vi "insert.vi"(8 "error in (no error)":errorcluster, 9 "Value":variant, 10 "Key":string, 11 "HashMap in":refnum<class "HashMap.lvclass">) -> (0 "error out":errorcluster, 3 "HashMap out":refnum<class "HashMap.lvclass">)   [LabVIEW 2017, in "HashMap.lvclass"]
uses:
  <userlib>/836-Library/Data_Structures/HashMap/HashMap.lvclass
  <userlib>/836-Library/Data_Structures/HashMap/HashMap.lvclass/HashMap.ctl
  <userlib>/836-Library/Data_Structures/Bucket/Types/KeyValuePair.ctl
  <vilib>/Utility/error.llb/Error Cluster From Error Code.vi
  <vilib>/ErrorRing/Error Ring.xnode
  <userlib>/836-Library/Data_Structures/Bucket/Bucket.lvclass
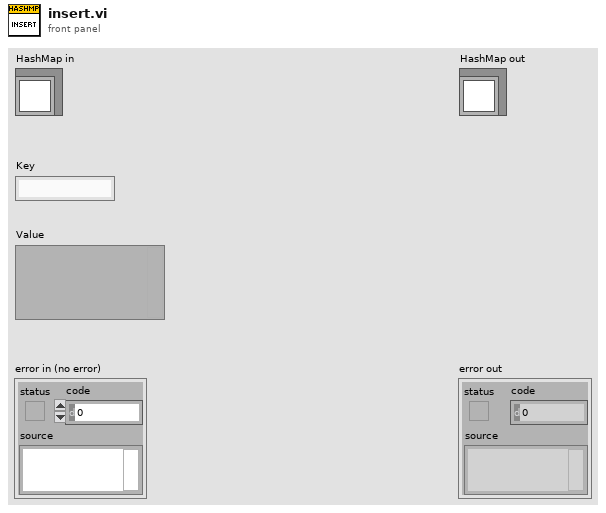
[diagram p1: front panel]
types:
  T1 = typedef "KeyValuePair.ctl" = cluster{"Key":string, "Value":variant}
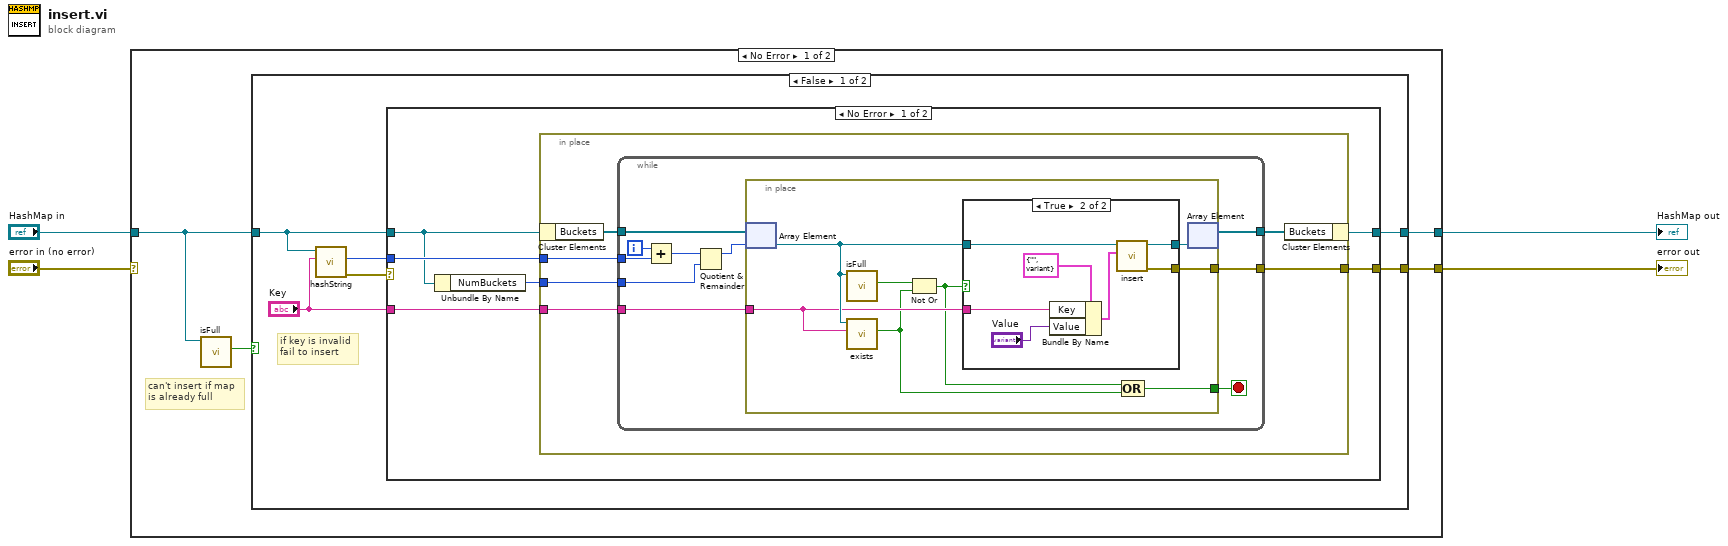
[diagram p0: block diagram]
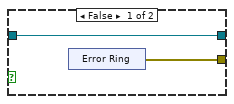
[diagram p2: hidden frame]
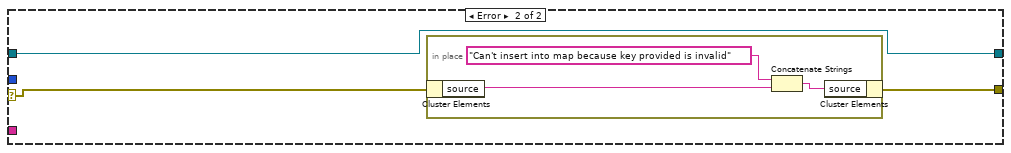
[diagram p3: hidden frame]
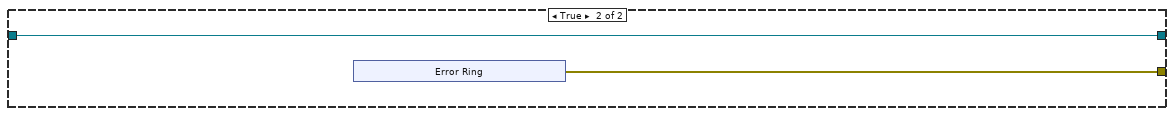
[diagram p4: hidden frame]
diagram:
  n1 = case shown="No Error" "error in (no error)" {
    selector: "error in (no error)" -> [_ w69]
    tunnel: [w6 w69] -> w3
    tunnel: [w5 w68] -> w1
    tunnel: "HashMap in" -> [w7 w68]
    frame No Error {
      # "can't insert if map\nis already full"
      n2 = call <userlib>:"isFull.vi"("HashMap in"=w7) -> ("Full?"=w8:bool)  [unwired: 8 in, 2 out]
      n3 = case shown="False" w8 {
        tunnel: w7 -> [w14 w61]
        tunnel: [w10 w62] -> w6
        tunnel: [w9 w61] -> w5
        frame False {
          # "if key is invalid\nfail to insert"
          n4 = call <userlib>:"hashString.vi"("String"="Key", "HashMap in"=w14) -> ("error out"=w12:errorcluster, "Hash"=w13:i32)  [unwired: 7 in, 1 out]
          n5 = case shown="No Error" w12 {
            selector: w12 -> [_ w57]
            tunnel: w14 -> [w19 w55]
            tunnel: w13 -> [w20 _]
            tunnel: "Key" -> [w17 _]
            tunnel: [w16 w56] -> w10
            tunnel: [w15 w55] -> w9
            frame No Error {
              n6 = Unbundle By Name(w19) -> ("NumBuckets"=w18:i32)
              n7 = in-place {
                in-place-border: w20 -> [w24]
                in-place-border: w18 -> [w23]
                in-place-border: w17 -> [w22]
                in-place-border: [w21] -> w16
                n8 = in-place-cluster #1(w19) -> ("Buckets"=w26:refnum<class "Bucket.lvclass">[])
                n9 = while {
                  tunnel: w26 -> [w35]
                  tunnel: [w36] -> w25
                  tunnel: w24 -> [w34]
                  tunnel: w23 -> [w29]
                  tunnel: w22 -> [w31]
                  tunnel: [w27] -> w21
                  i -> [w33]
                  stop <- w28 stop-if-true
                  n10 = Add(x=w33, y=w34) -> (x+y=w30:i32)
                  n11 = Quotient & Remainder(x=w30, y=w29) -> (x-y*floor(x/y)=w32:i32)  [unwired: 1 out]
                  n12 = in-place {
                    in-place-border: w31 -> [w43]
                    in-place-border: [w40] -> w28
                    in-place-border: [w38] -> w27
                    n13 = in-place-array #2(w35, w32) -> (w44:refnum<class "Bucket.lvclass">)
                    n14 = call <userlib>:"isFull.vi"("Bucket in"=w44) -> ("Full?"=w42:bool)  [unwired: 8 in, 2 out]
                    n15 = call <userlib>:"exists.vi"("Key"=w43, "Bucket in"=w44) -> ("Exists?"=w37:bool)  [unwired: 7 in, 2 out]
                    n16 = Not Or(1:w37, 2:w42) -> (0:w41:bool)
                    n17 = case shown="True" w41 {
                      tunnel: w44 -> [w46 w52]
                      tunnel: w43 -> [_ w50]
                      tunnel: [w46 w49] -> w39
                      tunnel: [w45 w48] -> w38
                      frame False {
                        n18 = xnode "Error Ring"() -> ("error out"=w45:errorcluster)
                      }
                      frame True {
                        n19 = Bundle By Name(cluster=T1 {"Key"="", "Value"=variant} ("To Insert"), "Key"=w50, "Value"="Value") -> (w53:T1)
                        n20 = call <userlib>:"insert.vi"("To Insert"=w53, "Bucket in"=w52) -> ("error out"=w48:errorcluster, "Bucket out"=w49:refnum<class "Bucket.lvclass">)  [unwired: 8 in]
                      }
                    }
                    n21 = Compound Arithmetic op=OR(w41, w37) -> (w40:bool)
                    n22 = in-place-array #2(w39) -> (w36:refnum<class "Bucket.lvclass">[])  [unwired: 1 out]
                  }
                }
                n23 = in-place-cluster #1("Buckets"=w25) -> (w15:refnum<class "HashMap.lvclass">)
              }
            }
            frame Error {
              n24 = in-place {
                n25 = in-place-cluster #3(w57) -> ("source"=w60:string)
                n26 = Concatenate Strings("Can't insert into map because key provided is invalid" ("string"), w60) -> (w58:string)
                n27 = in-place-cluster #3("source"=w58) -> (w56:errorcluster)
              }
            }
          }
        }
        frame True {
          n28 = xnode "Error Ring"() -> ("error out"=w62:errorcluster)
        }
      }
    }
    frame Error {
    }
  }
  "error out" <- w3
  "HashMap out" <- w1
